vi "activateCursor.vi"(8 "error in (no error)":errorcluster, 10 "Cursor On/Off":bool, 11 "dataClass in":refnum<class "SR430Class.lvclass">) -> (0 "error out":errorcluster, 3 "dataClass out":refnum<class "SR430Class.lvclass">)   [LabVIEW 2015, in "SR430Class.lvclass"]
uses:
  class/SR430Class.lvclass
  class/SR430Class.lvclass/SR430Class.ctl
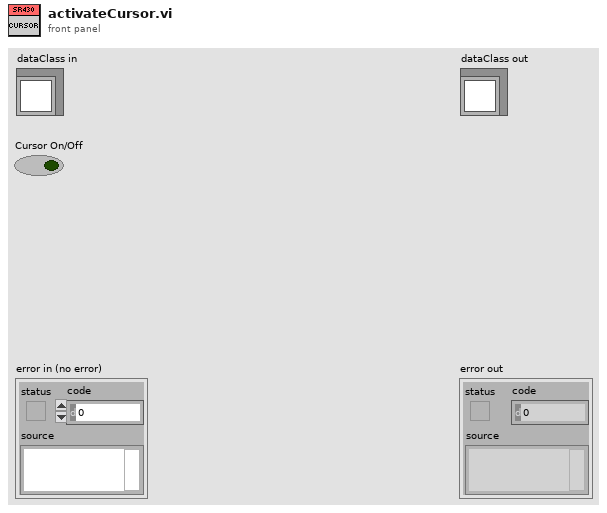
[diagram p1: front panel]
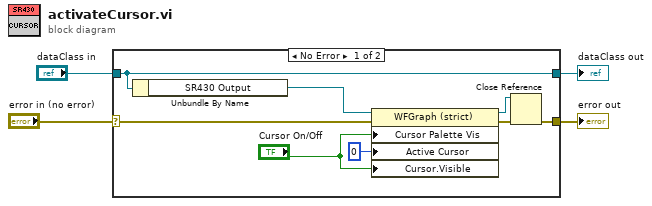
[diagram p0: block diagram]
diagram:
  n1 = case shown="No Error" "error in (no error)" {
    selector: "error in (no error)" -> [w10 w14]
    tunnel: [w7 w14] -> w3
    tunnel: [w12 w13] -> w1
    tunnel: "dataClass in" -> [w12 w13]
    frame No Error {
      n2 = Unbundle By Name(w12) -> ("SR430 Output"=w11:refnum<vi>)
      n3 = property on="Property Node" class="WFGraph (strict)"(reference=w11, error in=w10, "Cursor Palette Vis"="Cursor On/Off", "Active Cursor"=u32 0, "Cursor.Visible"="Cursor On/Off") -> (reference out=w9:refnum<vi>, error out=w8:errorcluster)
      n4 = Close Reference(reference=w9, error in (no error)=w8) -> (error out=w7:errorcluster)
    }
    frame Error {
    }
  }
  "error out" <- w3
  "dataClass out" <- w1
